vi "Actor Core.vi"(8 "error in":errorcluster, 11 "[V] Tester Parent in":refnum<class "[V] Tester Parent.lvclass">) -> (0 "error out":errorcluster, 3 "Actor out":refnum<class "Actor.lvclass">)   [LabVIEW 2020, in "[V] Tester Parent.lvlib" / "[V] Tester Parent.lvclass"]
doc: "(<B>Filename</B>: Actor Framework.lvlib:Actor.lvclass:Actor Core.vi)\n\nReceives messages to the actor, reacts to them, and initiates any error handling that may shut the actor down.\n\nDescendant classes may override this VI to append parallel tasks for the actor to complete while it handles messages. Overrides use the Call Parent Class Method node."
uses:
  [V] Tester Parent.lvclass
  D:/03 GitHub/LabVIEW-MDI-Panel/[MDI] Parent/[MDI] Parent/[MDI] Parent.lvclass
  C:/Program Files (x86)/National Instruments/LabVIEW 2020/vi.lib/ActorFramework/Actor/Actor.lvclass
  <vilib>/ActorFramework/Actor/Actor.lvclass
  <vilib>/ActorFramework/Actor/Actor.lvclass/Actor.ctl
  <vilib>/ActorFramework/Message Enqueuer/Message Enqueuer.lvclass/Message Enqueuer.ctl
  System.Drawing
  <vilib>/ActorFramework/Message Enqueuer/Init from Existing Queue.vi
  <vilib>/ActorFramework/Message Enqueuer/Enqueue.vi
  <vilib>/ActorFramework/Stop Msg/Stop Msg.lvclass
  C:/Program Files (x86)/National Instruments/LabVIEW 2020/vi.lib/ActorFramework/Message/Message.lvclass
  [V] Tester Parent Messages/Event New Child Msg/Event New Child Msg.lvclass
  [MDI] Parent/[MDI] Parent Messages/All Windows In Msg/All Windows In Msg.lvclass
  [MDI] Parent/[MDI] Parent Messages/All Windows Out Msg/All Windows Out Msg.lvclass
  [MDI] Parent/[MDI] Parent Messages/Arrange Cascade Msg/Arrange Cascade Msg.lvclass
  [MDI] Parent/[MDI] Parent Messages/Arrange Vertical Msg/Arrange Vertical Msg.lvclass
  [MDI] Parent/[MDI] Parent Messages/Arrange Horizontal Msg/Arrange Horizontal Msg.lvclass
  <vilib>/ActorFramework/Message Priority Queue/Priority Enqueue.vi
  <vilib>/ActorFramework/Message Enqueuer/Message Enqueuer.lvclass
  [MDI] Parent/[MDI] Parent/[MDI] Parent.lvclass
  System.Windows.Forms
panel:
  in  "out":bool
  in  "in":bool
  in  "cascade":bool
  in  "horizontal":bool
  in  "vertical":bool
  in  "new child":bool
  in  "parent panel":refnum<k24>(container)
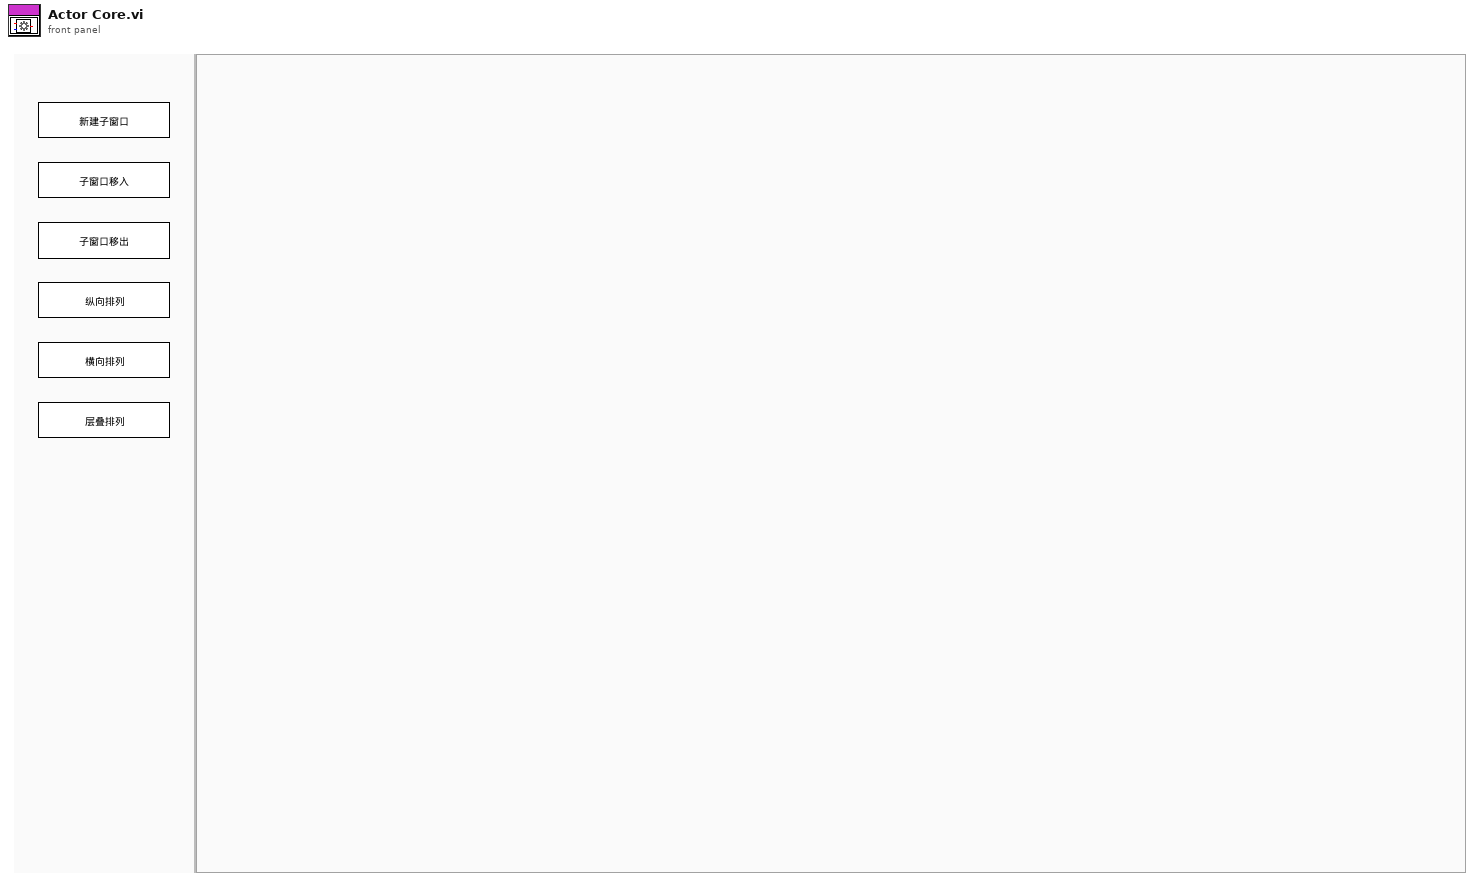
[diagram p1: front panel]
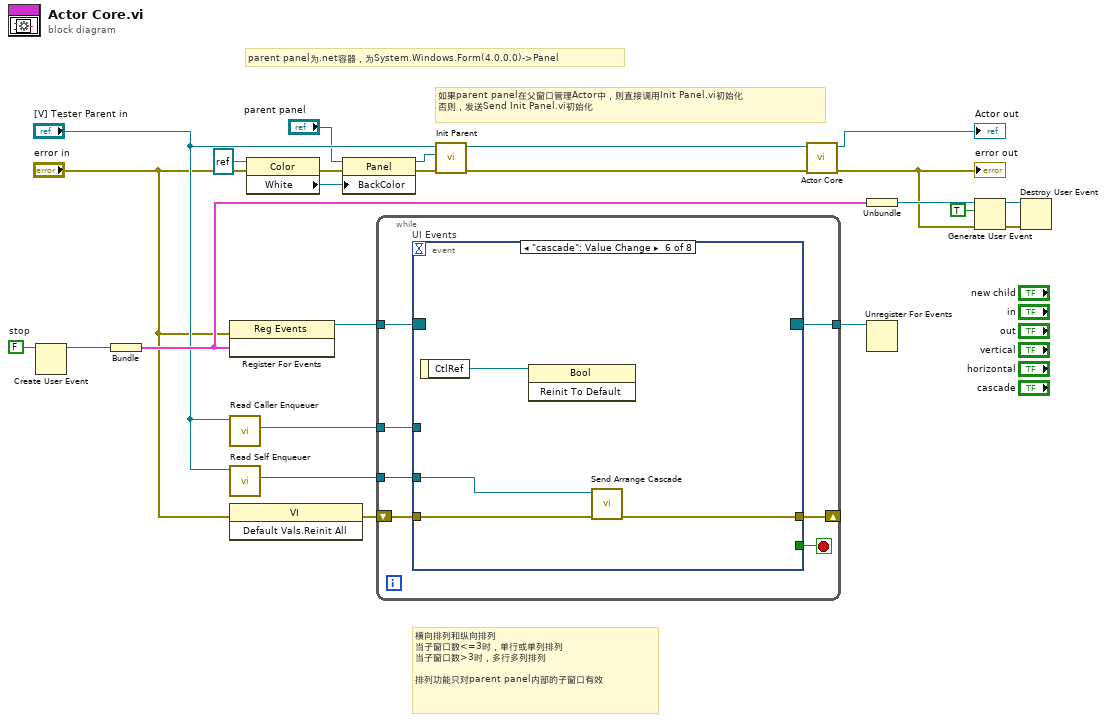
[diagram p0: block diagram]
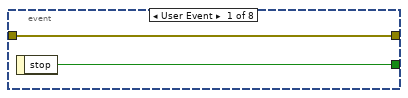
[diagram p2: hidden frame]
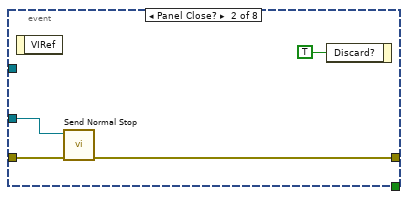
[diagram p3: hidden frame]
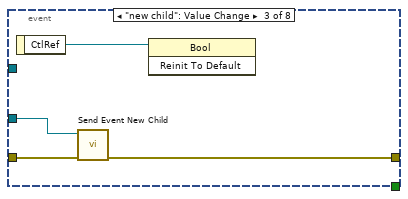
[diagram p4: hidden frame]
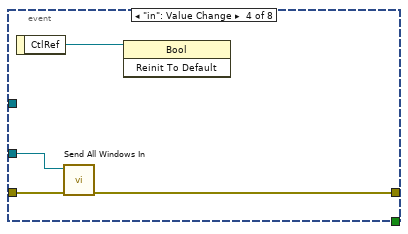
[diagram p5: hidden frame]
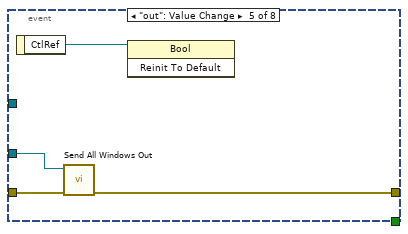
[diagram p6: hidden frame]
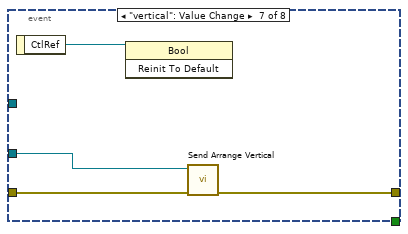
[diagram p7: hidden frame]
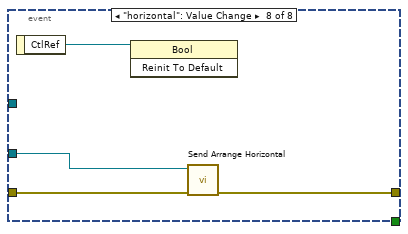
[diagram p8: hidden frame]
diagram:
  w17 = FALSE  # stop
  # "横向排列和纵向排列\n当子窗口数<=3时，单行或单列排列\n当子窗口数>3时，多行多列排列\n\n排列功能只对parent panel内部的子窗口有效"
  # "如果parent panel在父窗口管理Actor中，则直接调用Init Panel.vi初始化\n否则，发送Send Init Panel.vi初始化"
  # "parent panel为.net容器，为System.Windows.Form(4.0.0.0)->Panel"
  n1 = Create User Event(user event datatype=w17) -> (user event=w20:refnum<user-event>)  [unwired: 1 in, 1 out]
  n2 = Bundle("stop"=w20) -> (w21:cluster{"stop":refnum<user-event>})  [unwired: 1 in]
  n3 = register-events ("Main Register for Events")(error in="error in", w21) -> (reference out=w12:refnum<event-registration>)  [unwired: 1 in, 1 out]
  n4 = call <vilib>:"Read Caller Enqueuer.vi"("Actor"="[V] Tester Parent in") -> ("Caller Enqueuer"=w15:refnum<class "Message Enqueuer.lvclass">)  [unwired: 10 in]
  n5 = call <vilib>:"Read Self Enqueuer.vi"("Actor"="[V] Tester Parent in") -> ("Self Enqueuer"=w14:refnum<class "Message Enqueuer.lvclass">)  [unwired: 10 in]
  n6 = invoke class="VI" method="Default Vals.Reinit All"(error in="error in") -> (error out=w16:errorcluster)  [unwired: 2 in, 2 out]
  n7 = property class="Color"(reference=refnum<k24> refnum ("BackColor"), error in="error in") -> (error out=w5:errorcluster, "White"=w4:refnum<k24>)  [unwired: 1 out]
  n8 = property class="Panel"(reference="parent panel", error in=w5, "BackColor"=w4) -> (reference out=w1:refnum<k24>, error out=w2:errorcluster)
  n9 = while {
    tunnel: w12 -> [w31]
    tunnel: [w29] -> w13
    tunnel: w14 -> [w28]
    tunnel: w15 -> [w25]
    shift-right: [w26] -> _
    shift-left: w16 -> [w27]
    stop <- w30 stop-if-true
    n10 = event "UI Events" shown="[5] \"cascade\": Value Change" {
      selector: w31 -> [_ _ _ _ _ _ _ _]
      dyn-events: [_ _ _ _ _ _ _ _] -> w29
      timeout: _ -> [_ _ _ _ _ _ _ _]
      tunnel: [w32 _ _ _ _ _ _ _] -> w30
      tunnel: w28 -> [_ w36 w40 w44 w48 w51 w55 w59]
      tunnel: w27 -> [w33 w35 w41 w45 w49 w53 w57 w61]
      tunnel: [w33 w34 w39 w43 w47 w52 w56 w60] -> w26
      tunnel: w25 -> [_ _ _ _ _ _ _ _]
      event User Event {
        n11 = event-data() -> ("stop"=w32:bool)  [unwired: 1 in]
      }
      event Panel Close? {
        n12 = event-data() -> ()  [unwired: 1 in, 1 out]
        n13 = call <vilib>:"Send Normal Stop.vi"("error in (no error)"=w35, "Message Enqueuer"=w36) -> ("error out"=w34:errorcluster)  [unwired: 9 in]
        n14 = event-data("Discard?"=TRUE) -> ()  [unwired: 1 in, 1 out]
      }
      event "new child": Value Change {
        n15 = event-data() -> ("CtlRef"=w38:refnum<vi>)  [unwired: 1 in]
        n16 = call "Send Event New Child.vi"("error in (no error)"=w41, "Message Enqueuer"=w40) -> ("error out"=w39:errorcluster)  [unwired: 8 in, 1 out]
        n17 = invoke class="Bool" method="Reinit To Default"(reference=w38) -> ()  [unwired: 2 in, 3 out]
      }
      event "in": Value Change {
        n18 = event-data() -> ("CtlRef"=w42:refnum<vi>)  [unwired: 1 in]
        n19 = call "Send All Windows In.vi"("error in (no error)"=w45, "Message Enqueuer"=w44) -> ("error out"=w43:errorcluster)  [unwired: 8 in, 1 out]
        n20 = invoke class="Bool" method="Reinit To Default"(reference=w42) -> ()  [unwired: 2 in, 3 out]
      }
      event "out": Value Change {
        n21 = event-data() -> ("CtlRef"=w46:refnum<vi>)  [unwired: 1 in]
        n22 = call "Send All Windows Out.vi"("error in (no error)"=w49, "Message Enqueuer"=w48) -> ("error out"=w47:errorcluster)  [unwired: 8 in, 1 out]
        n23 = invoke class="Bool" method="Reinit To Default"(reference=w46) -> ()  [unwired: 2 in, 3 out]
      }
      event "cascade": Value Change {
        n24 = event-data() -> ("CtlRef"=w50:refnum<vi>)  [unwired: 1 in]
        n25 = invoke class="Bool" method="Reinit To Default"(reference=w50) -> ()  [unwired: 2 in, 3 out]
        n26 = call "Send Arrange Cascade.vi"("error in (no error)"=w53, "Message Enqueuer"=w51) -> ("error out"=w52:errorcluster)  [unwired: 8 in, 1 out]
      }
      event "vertical": Value Change {
        n27 = event-data() -> ("CtlRef"=w54:refnum<vi>)  [unwired: 1 in]
        n28 = invoke class="Bool" method="Reinit To Default"(reference=w54) -> ()  [unwired: 2 in, 3 out]
        n29 = call "Send Arrange Vertical.vi"("error in (no error)"=w57, "Message Enqueuer"=w55) -> ("error out"=w56:errorcluster)  [unwired: 8 in, 1 out]
      }
      event "horizontal": Value Change {
        n30 = event-data() -> ("CtlRef"=w58:refnum<vi>)  [unwired: 1 in]
        n31 = invoke class="Bool" method="Reinit To Default"(reference=w58) -> ()  [unwired: 2 in, 3 out]
        n32 = call "Send Arrange Horizontal.vi"("error in (no error)"=w61, "Message Enqueuer"=w59) -> ("error out"=w60:errorcluster)  [unwired: 8 in, 1 out]
      }
    }
  }
  n33 = call "Init Parent.vi"("error in (no error)"=w2, ".net panel"=w1, "[MDI] Parent in"="[V] Tester Parent in") -> ("error out"=w9:errorcluster, "[MDI] Parent out"=w8:refnum<class "[V] Tester Parent.lvclass">)  [unwired: 7 in]
  n34 = call-parent "Actor Core.vi"("error in"=w9, "Actor in"=w8) -> ("error out"=w11:errorcluster, "Actor out"=→"Actor out":refnum<class "Actor.lvclass">)  [unwired: 8 in]
  "error out" <- w11
  n35 = Unbundle(w21) -> ("stop"=w22:refnum<user-event>)
  n36 = Unregister For Events(event registration refnum=w13) -> ()  [unwired: 1 in, 1 out]
  n37 = Generate User Event(user event=w22, event data cluster=TRUE ("event data"), error in=w11) -> (user event out=w19:refnum<user-event>, error out=w23:errorcluster)  [unwired: 1 in]
  n38 = Destroy User Event(user event=w19, error in=w23) -> ()  [unwired: 1 out]
